vi "5T_open_queue.vi"(8 "error in (no error)":errorcluster) -> (0 "error out":errorcluster, 2 "queue out":refnum<queue>)   [LabVIEW 2019]
uses:
  Mischer/5T-Cluster.ctl
  Global/Global Variables/Queues_global.vi
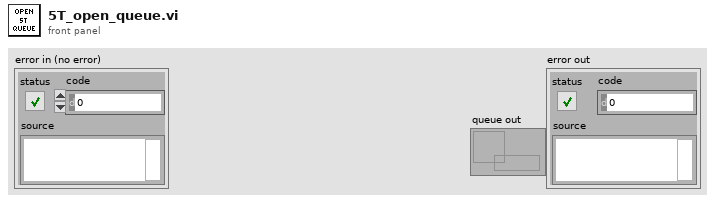
[diagram p1: front panel]
types:
  T1 = typedef "5T-Cluster.ctl" = cluster{"Go to set":bool, "Go to Zero":bool, "Clamp":bool, "Go to Hold":bool, "Clamped ":bool, "Quenched 2":bool, "Rate limit 2":bool, "Magnet (T)":dbl, "Leads (T)":dbl, "Rate (T/min)":dbl, "Sweeping":bool, "Setpoint":dbl, "Set":bool, "Zero":bool, "Hold":bool, "Clamp":bool}
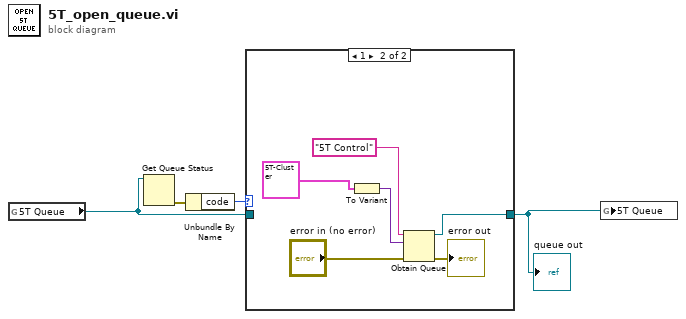
[diagram p0: block diagram]
diagram:
  n1 = global read "Queues_global.vi" "5T Queue"() -> (w2:refnum<queue>)
  n2 = Get Queue Status(queue=w2) -> (error out=w4:errorcluster)  [unwired: 2 in, 7 out]
  n3 = Unbundle By Name(w4) -> ("code"=w3:i32)
  n4 = case shown="1" w3 {
    tunnel: [w5 w7] -> w1
    tunnel: w2 -> [w5 _]
    frame 0, Default {
    }
    frame 1 {
      n5 = To Variant(anything=T1 {"Go to set"=FALSE, "Go to Zero"=FALSE, "Clamp"=FALSE, "Go to Hold"=FALSE, "Clamped "=FALSE, "Quenched 2"=FALSE, "Rate limit 2"=FALSE, "Magnet (T)"=0.0, "Leads (T)"=0.0, "Rate (T/min)"=0.0, "Sweeping"=FALSE, "Setpoint"=0.0, "Set"=FALSE, "Zero"=FALSE, "Hold"=FALSE, "Clamp"=FALSE} ("5 T Cluster")) -> (Variant=w10:variant)
      n6 = Obtain Queue(name (unnamed)="5T Control", element data type=w10, error in (no error)="error in (no error)") -> (queue out=w7:refnum<queue>, error out=→"error out":errorcluster)  [unwired: 2 in, 1 out]
    }
  }
  "queue out" <- w1
  n7 = global write "Queues_global.vi" "5T Queue"(w1) -> ()
